vi "PRUEBA_Serial_v0.2.vi"() -> ()   [LabVIEW 2011]
panel:
  in  "SON":bool
  in  "Direccion":bool
  in  "Fout":u32(slide) scale=0.0..100000.0
  in  "Vout":dbl(slide) scale=-10.0..10.0
  in  "VISA COM IN":refnum<visa-resource-name>
  in  "stop":bool
  # "Prueba de Comunicacion Serial - Deslizador"
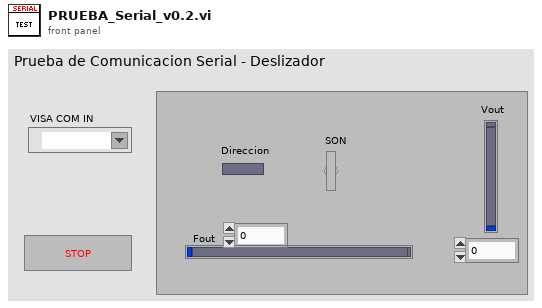
[diagram p1: front panel]
types:
  T1 = enum16{"Aout", "Fout", "Direccion", "ServoOn", "Idle"}
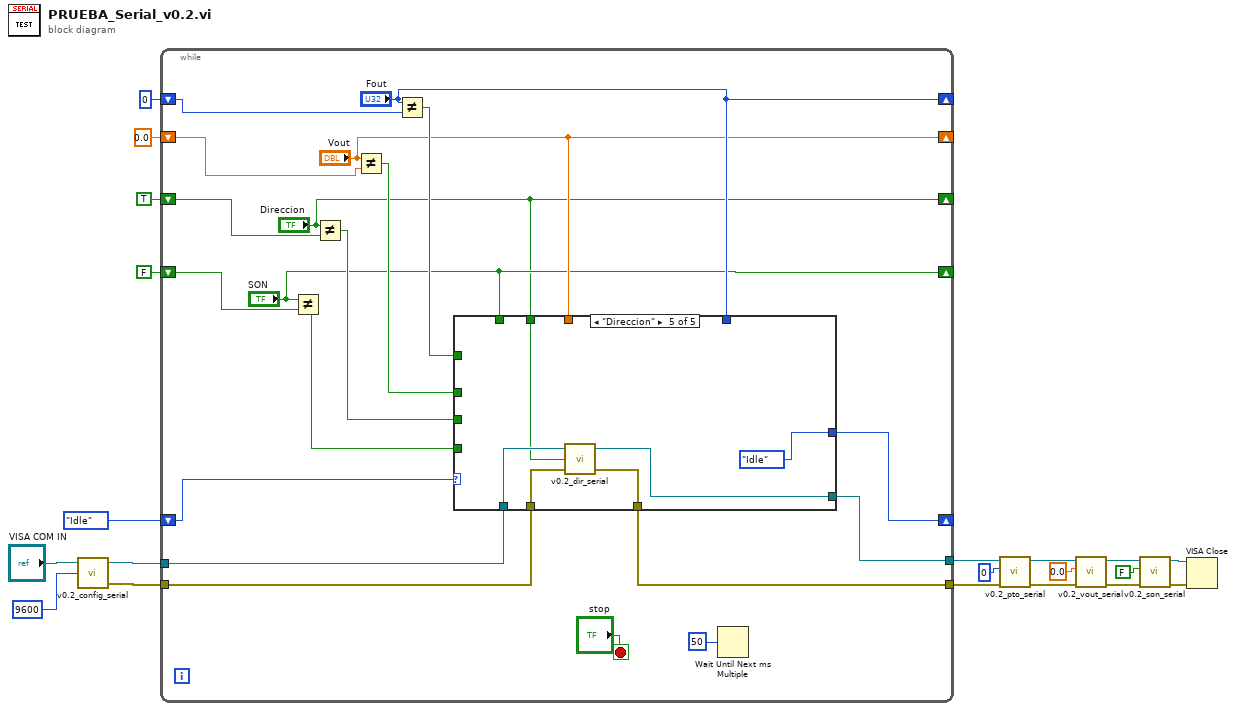
[diagram p0: block diagram]
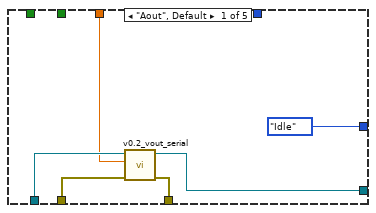
[diagram p2: hidden frame]
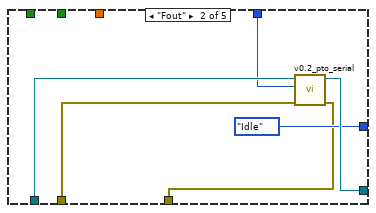
[diagram p3: hidden frame]
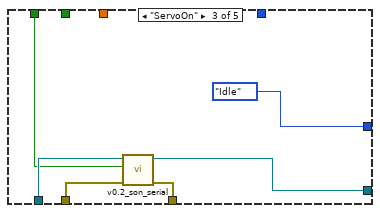
[diagram p4: hidden frame]
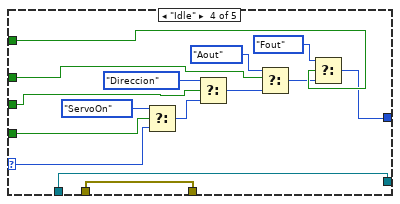
[diagram p5: hidden frame]
diagram:
  n1 = call "v0.2_config_serial.vi"("baud rate (9600/115200)"=u32 9600, "VISA COM IN"="VISA COM IN") -> ("error out"=w18:errorcluster, "VISA COM OUT"=w19:refnum<visa-resource-name>)  [unwired: 2 in]
  n2 = while {
    tunnel: w19 -> [w28]
    tunnel: w18 -> [w22]
    shift-right: ["Fout"] -> _
    shift-left: u32 0 ("Fout") -> [w39]
    shift-right: ["Vout"] -> _
    shift-left: 0.0 ("Volt") -> [w38]
    tunnel: [w21] -> w8
    shift-right: [w33] -> _
    shift-left: T1."Idle" -> [w36]
    shift-right: ["Direccion"] -> _
    shift-left: TRUE ("Direccion") -> [w32]
    shift-right: ["SON"] -> _
    shift-left: FALSE ("SON") -> [w30]
    tunnel: [w26] -> w12
    stop <- "stop" stop-if-true
    n3 = Not Equal?(x="SON", y=w30) -> (x != y?=w29:bool)
    n4 = Not Equal?(x="Direccion", y=w32) -> (x != y?=w31:bool)
    n5 = Not Equal?(x="Vout", y=w38) -> (x != y?=w35:bool)
    n6 = Not Equal?(x="Fout", y=w39) -> (x != y?=w34:bool)
    n7 = case shown="\"Direccion\"" w36 {
      selector: w36 -> [_ _ _ w63 _]
      tunnel: w35 -> [_ _ _ w71 _]
      tunnel: w34 -> [_ _ _ w73 _]
      tunnel: [T1."Idle" T1."Idle" T1."Idle" w68 T1."Idle"] -> w33
      tunnel: w31 -> [_ _ _ w61 _]
      tunnel: w29 -> [_ _ _ w62 _]
      tunnel: w28 -> [w46 w52 w58 w60 w79]
      tunnel: "Fout" -> [_ w51 _ _ _]
      tunnel: [w44 w50 w56 w60 w77] -> w26
      tunnel: "Vout" -> [w45 _ _ _ _]
      tunnel: "SON" -> [_ _ w57 _ _]
      tunnel: "Direccion" -> [_ _ _ _ w78]
      tunnel: w22 -> [w42 w48 w54 w59 w75]
      tunnel: [w41 w47 w53 w59 w74] -> w21
      frame "Aout", Default {
        n8 = call "v0.2_vout_serial.vi"("error in (no error)"=w42, "Volt"=w45, "VISA COM IN"=w46) -> ("error out"=w41:errorcluster, "VISA COM OUT"=w44:refnum<visa-resource-name>)  [unwired: 7 in]
      }
      frame "Fout" {
        n9 = call "v0.2_pto_serial.vi"("error in (no error)"=w48, "Fout"=w51, "VISA COM IN"=w52) -> ("error out"=w47:errorcluster, "VISA COM OUT"=w50:refnum<visa-resource-name>)  [unwired: 7 in]
      }
      frame "ServoOn" {
        n10 = call "v0.2_son_serial.vi"("error in (no error)"=w54, "ServoON"=w57, "VISA COM IN"=w58) -> ("error out"=w53:errorcluster, "VISA COM OUT"=w56:refnum<visa-resource-name>)  [unwired: 7 in]
      }
      frame "Idle" {
        n11 = Select(t=T1."ServoOn", s=w62, f=w63) -> (s? t:f=w64:T1)
        n12 = Select(t=T1."Direccion", s=w61, f=w64) -> (s? t:f=w65:T1)
        n13 = Select(t=T1."Aout", s=w71, f=w65) -> (s? t:f=w69:T1)
        n14 = Select(t=T1."Fout", s=w73, f=w69) -> (s? t:f=w68:T1)
      }
      frame "Direccion" {
        n15 = call "v0.2_dir_serial.vi"("error in (no error)"=w75, "Direccion"=w78, "VISA COM IN"=w79) -> ("error out"=w74:errorcluster, "VISA COM OUT"=w77:refnum<visa-resource-name>)  [unwired: 1 in]
      }
    }
    n16 = Wait Until Next ms Multiple(millisecond multiple=u32 50) -> ()  [unwired: 1 out]
  }
  n17 = call "v0.2_pto_serial.vi"("error in (no error)"=w8, "Fout"=u32 0, "VISA COM IN"=w12) -> ("error out"=w7:errorcluster, "VISA COM OUT"=w11:refnum<visa-resource-name>)  [unwired: 7 in]
  n18 = call "v0.2_vout_serial.vi"("error in (no error)"=w7, "Volt"=0.0, "VISA COM IN"=w11) -> ("error out"=w6:errorcluster, "VISA COM OUT"=w10:refnum<visa-resource-name>)  [unwired: 7 in]
  n19 = call "v0.2_son_serial.vi"("error in (no error)"=w6, "ServoON"=FALSE, "VISA COM IN"=w10) -> ("error out"=w5:errorcluster, "VISA COM OUT"=w9:refnum<visa-resource-name>)  [unwired: 7 in]
  n20 = VISA Close(VISA resource name=w9, error in (no error)=w5) -> ()  [unwired: 1 out]
